vi "CheckInterlocking.vi"() -> (0 "All_Interlock":bool[](array[boolean]), 1 "AllExcept0":bool, 2 "ALL":bool, 3 "Only_0":bool)   [LabVIEW 2020]
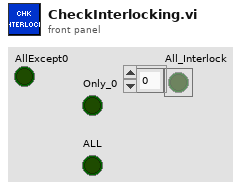
[diagram p1: front panel]
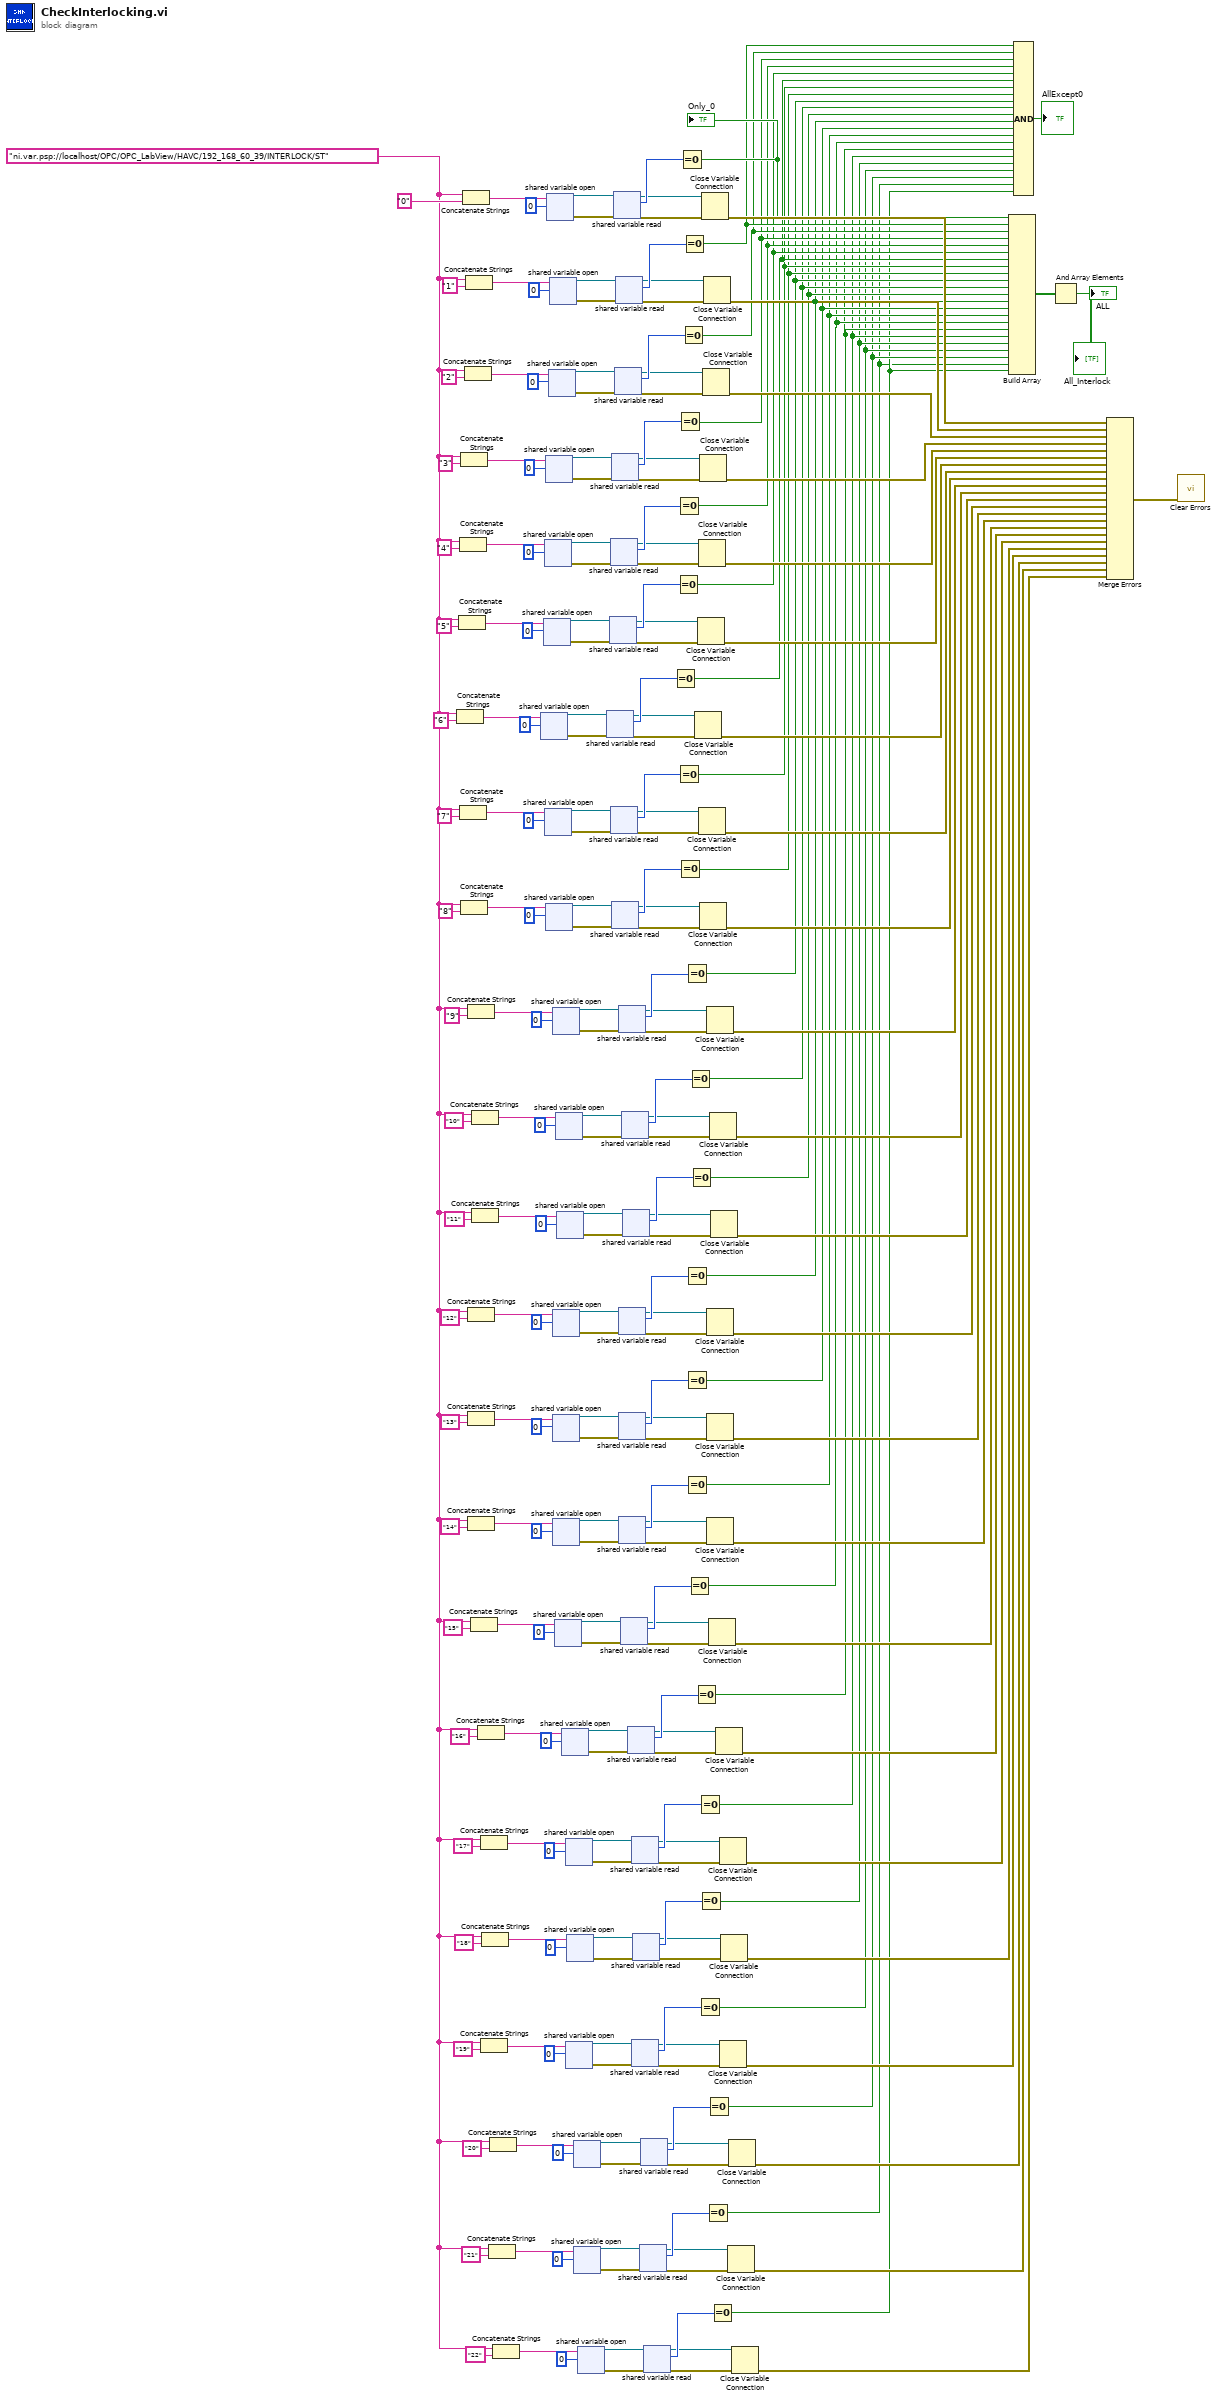
[diagram p0: block diagram]
diagram:
  w29 = "ni.var.psp://localhost/OPC/OPC_LabView/HAVC/192_168_60_39/INTERLOCK/ST" ("string")
  n1 = Concatenate Strings(w29, "6" ("string")) -> (w189:string)
  n2 = Concatenate Strings(w29, "5" ("string")) -> (w196:string)
  n3 = Concatenate Strings(w29, "4" ("string")) -> (w203:string)
  n4 = Concatenate Strings(w29, "7" ("string")) -> (w182:string)
  n5 = Concatenate Strings(w29, "3" ("string")) -> (w210:string)
  n6 = Concatenate Strings(w29, "8" ("string")) -> (w175:string)
  n7 = Concatenate Strings(w29, "0" ("string")) -> (w231:string)
  n8 = Concatenate Strings(w29, "2" ("string")) -> (w217:string)
  n9 = Concatenate Strings(w29, "1" ("string")) -> (w224:string)
  n10 = Concatenate Strings(w29, "9" ("string")) -> (w168:string)
  n11 = Concatenate Strings(w29, "12" ("string")) -> (w147:string)
  n12 = Concatenate Strings(w29, "13" ("string")) -> (w140:string)
  n13 = Concatenate Strings(w29, "14" ("string")) -> (w133:string)
  n14 = Concatenate Strings(w29, "15" ("string")) -> (w126:string)
  n15 = Concatenate Strings(w29, "10" ("string")) -> (w161:string)
  n16 = Concatenate Strings(w29, "11" ("string")) -> (w154:string)
  n17 = Concatenate Strings(w29, "16" ("string")) -> (w119:string)
  n18 = Concatenate Strings(w29, "17" ("string")) -> (w112:string)
  n19 = Concatenate Strings(w29, "19" ("string")) -> (w98:string)
  n20 = Concatenate Strings(w29, "18" ("string")) -> (w105:string)
  n21 = Concatenate Strings(w29, "21" ("string")) -> (w84:string)
  n22 = Concatenate Strings(w29, "20" ("string")) -> (w91:string)
  n23 = Concatenate Strings(w29, "22" ("string")) -> (w77:string)
  n24 = shared-variable-open(w189, 0) -> (w190:refnum<k21>, w191:errorcluster)  [unwired: 2 in]
  n25 = shared-variable-open(w196, 0) -> (w197:refnum<k21>, w198:errorcluster)  [unwired: 2 in]
  n26 = shared-variable-open(w203, 0) -> (w204:refnum<k21>, w205:errorcluster)  [unwired: 2 in]
  n27 = shared-variable-open(w182, 0) -> (w183:refnum<k21>, w184:errorcluster)  [unwired: 2 in]
  n28 = shared-variable-open(w210, 0) -> (w211:refnum<k21>, w212:errorcluster)  [unwired: 2 in]
  n29 = shared-variable-open(w175, 0) -> (w176:refnum<k21>, w177:errorcluster)  [unwired: 2 in]
  n30 = shared-variable-open(w231, 0) -> (w232:refnum<k21>, w233:errorcluster)  [unwired: 2 in]
  n31 = shared-variable-open(w217, 0) -> (w218:refnum<k21>, w219:errorcluster)  [unwired: 2 in]
  n32 = shared-variable-open(w224, 0) -> (w225:refnum<k21>, w226:errorcluster)  [unwired: 2 in]
  n33 = shared-variable-open(w168, 0) -> (w169:refnum<k21>, w170:errorcluster)  [unwired: 2 in]
  n34 = shared-variable-open(w147, 0) -> (w148:refnum<k21>, w149:errorcluster)  [unwired: 2 in]
  n35 = shared-variable-open(w140, 0) -> (w141:refnum<k21>, w142:errorcluster)  [unwired: 2 in]
  n36 = shared-variable-open(w133, 0) -> (w134:refnum<k21>, w135:errorcluster)  [unwired: 2 in]
  n37 = shared-variable-open(w126, 0) -> (w127:refnum<k21>, w128:errorcluster)  [unwired: 2 in]
  n38 = shared-variable-open(w161, 0) -> (w162:refnum<k21>, w163:errorcluster)  [unwired: 2 in]
  n39 = shared-variable-open(w154, 0) -> (w155:refnum<k21>, w156:errorcluster)  [unwired: 2 in]
  n40 = shared-variable-open(w119, 0) -> (w120:refnum<k21>, w121:errorcluster)  [unwired: 2 in]
  n41 = shared-variable-open(w112, 0) -> (w113:refnum<k21>, w114:errorcluster)  [unwired: 2 in]
  n42 = shared-variable-open(w98, 0) -> (w99:refnum<k21>, w100:errorcluster)  [unwired: 2 in]
  n43 = shared-variable-open(w105, 0) -> (w106:refnum<k21>, w107:errorcluster)  [unwired: 2 in]
  n44 = shared-variable-open(w84, 0) -> (w85:refnum<k21>, w86:errorcluster)  [unwired: 2 in]
  n45 = shared-variable-open(w91, 0) -> (w92:refnum<k21>, w93:errorcluster)  [unwired: 2 in]
  n46 = shared-variable-open(w77, 0) -> (w78:refnum<k21>, w79:errorcluster)  [unwired: 2 in]
  n47 = shared-variable-read(w190, w191) -> (w186:refnum<k21>, w187:errorcluster, w188:i32)  [unwired: 1 out]
  n48 = shared-variable-read(w197, w198) -> (w193:refnum<k21>, w194:errorcluster, w195:i32)  [unwired: 1 out]
  n49 = shared-variable-read(w204, w205) -> (w200:refnum<k21>, w201:errorcluster, w202:i32)  [unwired: 1 out]
  n50 = shared-variable-read(w183, w184) -> (w179:refnum<k21>, w180:errorcluster, w181:i32)  [unwired: 1 out]
  n51 = shared-variable-read(w211, w212) -> (w207:refnum<k21>, w208:errorcluster, w209:i32)  [unwired: 1 out]
  n52 = shared-variable-read(w176, w177) -> (w172:refnum<k21>, w173:errorcluster, w174:i32)  [unwired: 1 out]
  n53 = shared-variable-read(w232, w233) -> (w228:refnum<k21>, w229:errorcluster, w230:i32)  [unwired: 1 out]
  n54 = shared-variable-read(w218, w219) -> (w214:refnum<k21>, w215:errorcluster, w216:i32)  [unwired: 1 out]
  n55 = shared-variable-read(w225, w226) -> (w221:refnum<k21>, w222:errorcluster, w223:i32)  [unwired: 1 out]
  n56 = shared-variable-read(w169, w170) -> (w165:refnum<k21>, w166:errorcluster, w167:i32)  [unwired: 1 out]
  n57 = shared-variable-read(w148, w149) -> (w144:refnum<k21>, w145:errorcluster, w146:i32)  [unwired: 1 out]
  n58 = shared-variable-read(w141, w142) -> (w137:refnum<k21>, w138:errorcluster, w139:i32)  [unwired: 1 out]
  n59 = shared-variable-read(w134, w135) -> (w130:refnum<k21>, w131:errorcluster, w132:i32)  [unwired: 1 out]
  n60 = shared-variable-read(w127, w128) -> (w123:refnum<k21>, w124:errorcluster, w125:i32)  [unwired: 1 out]
  n61 = shared-variable-read(w162, w163) -> (w158:refnum<k21>, w159:errorcluster, w160:i32)  [unwired: 1 out]
  n62 = shared-variable-read(w155, w156) -> (w151:refnum<k21>, w152:errorcluster, w153:i32)  [unwired: 1 out]
  n63 = shared-variable-read(w120, w121) -> (w116:refnum<k21>, w117:errorcluster, w118:i32)  [unwired: 1 out]
  n64 = shared-variable-read(w113, w114) -> (w109:refnum<k21>, w110:errorcluster, w111:i32)  [unwired: 1 out]
  n65 = shared-variable-read(w99, w100) -> (w95:refnum<k21>, w96:errorcluster, w97:i32)  [unwired: 1 out]
  n66 = shared-variable-read(w106, w107) -> (w102:refnum<k21>, w103:errorcluster, w104:i32)  [unwired: 1 out]
  n67 = shared-variable-read(w85, w86) -> (w81:refnum<k21>, w82:errorcluster, w83:i32)  [unwired: 1 out]
  n68 = shared-variable-read(w92, w93) -> (w88:refnum<k21>, w89:errorcluster, w90:i32)  [unwired: 1 out]
  n69 = shared-variable-read(w78, w79) -> (w74:refnum<k21>, w75:errorcluster, w76:i32)  [unwired: 1 out]
  n70 = Equal To 0?(x=w188) -> (x = 0?=w19:bool)
  n71 = Equal To 0?(x=w195) -> (x = 0?=w20:bool)
  n72 = Equal To 0?(x=w202) -> (x = 0?=w21:bool)
  n73 = Equal To 0?(x=w181) -> (x = 0?=w18:bool)
  n74 = Equal To 0?(x=w209) -> (x = 0?=w22:bool)
  n75 = Equal To 0?(x=w174) -> (x = 0?=w17:bool)
  n76 = Equal To 0?(x=w230) -> (x = 0?=w26:bool)
  "Only_0" <- w26
  n77 = Equal To 0?(x=w216) -> (x = 0?=w24:bool)
  n78 = Equal To 0?(x=w223) -> (x = 0?=w25:bool)
  n79 = Equal To 0?(x=w167) -> (x = 0?=w16:bool)
  n80 = Equal To 0?(x=w146) -> (x = 0?=w13:bool)
  n81 = Equal To 0?(x=w139) -> (x = 0?=w12:bool)
  n82 = Equal To 0?(x=w132) -> (x = 0?=w11:bool)
  n83 = Equal To 0?(x=w125) -> (x = 0?=w10:bool)
  n84 = Equal To 0?(x=w160) -> (x = 0?=w15:bool)
  n85 = Equal To 0?(x=w153) -> (x = 0?=w14:bool)
  n86 = Equal To 0?(x=w118) -> (x = 0?=w9:bool)
  n87 = Close Variable Connection(8:w187, 11:w186) -> (0:w64:errorcluster)
  n88 = Equal To 0?(x=w111) -> (x = 0?=w8:bool)
  n89 = Equal To 0?(x=w97) -> (x = 0?=w6:bool)
  n90 = Close Variable Connection(8:w194, 11:w193) -> (0:w65:errorcluster)
  n91 = Equal To 0?(x=w104) -> (x = 0?=w7:bool)
  n92 = Close Variable Connection(8:w201, 11:w200) -> (0:w66:errorcluster)
  n93 = Close Variable Connection(8:w180, 11:w179) -> (0:w63:errorcluster)
  n94 = Close Variable Connection(8:w208, 11:w207) -> (0:w67:errorcluster)
  n95 = Close Variable Connection(8:w173, 11:w172) -> (0:w62:errorcluster)
  n96 = Close Variable Connection(8:w229, 11:w228) -> (0:w70:errorcluster)
  n97 = Close Variable Connection(8:w215, 11:w214) -> (0:w68:errorcluster)
  n98 = Close Variable Connection(8:w222, 11:w221) -> (0:w69:errorcluster)
  n99 = Equal To 0?(x=w83) -> (x = 0?=w3:bool)
  n100 = Equal To 0?(x=w90) -> (x = 0?=w5:bool)
  n101 = Close Variable Connection(8:w166, 11:w165) -> (0:w61:errorcluster)
  n102 = Close Variable Connection(8:w145, 11:w144) -> (0:w58:errorcluster)
  n103 = Close Variable Connection(8:w138, 11:w137) -> (0:w57:errorcluster)
  n104 = Close Variable Connection(8:w131, 11:w130) -> (0:w56:errorcluster)
  n105 = Close Variable Connection(8:w124, 11:w123) -> (0:w55:errorcluster)
  n106 = Equal To 0?(x=w76) -> (x = 0?=w4:bool)
  n107 = Close Variable Connection(8:w159, 11:w158) -> (0:w60:errorcluster)
  n108 = Close Variable Connection(8:w152, 11:w151) -> (0:w59:errorcluster)
  n109 = Close Variable Connection(8:w117, 11:w116) -> (0:w54:errorcluster)
  n110 = Close Variable Connection(8:w110, 11:w109) -> (0:w53:errorcluster)
  n111 = Close Variable Connection(8:w96, 11:w95) -> (0:w51:errorcluster)
  n112 = Close Variable Connection(8:w103, 11:w102) -> (0:w52:errorcluster)
  n113 = Close Variable Connection(8:w82, 11:w81) -> (0:w49:errorcluster)
  n114 = Close Variable Connection(8:w89, 11:w88) -> (0:w50:errorcluster)
  n115 = Close Variable Connection(8:w75, 11:w74) -> (0:w48:errorcluster)
  n116 = Build Array(w26, w25, w24, w22, w21, w20, w19, w18, w17, w16, w15, w14, w13, w12, w11, w10, w9, w8, w7, w6, w5, w3, w4) -> (w1:bool[])
  "All_Interlock" <- w1
  n117 = Compound Arithmetic op=AND(w25, w24, w22, w21, w20, w19, w18, w17, w16, w15, w14, w13, w12, w11, w10, w9, w8, w7, w6, w5, w3, w4) -> (→"AllExcept0":bool)
  n118 = And Array Elements(Boolean array=w1) -> (logical AND=→"ALL":bool)
  n119 = Merge Errors(w70, w69, w68, w67, w66, w65, w64, w63, w62, w61, w60, w59, w58, w57, w56, w55, w54, w53, w52, w51, w50, w49, w48) -> (w47:errorcluster)
  n120 = call <vilib>:"Clear Errors.vi"("error in (no error)"=w47) -> ()  [unwired: 5 in, 2 out]
